vi "Append Ring StringsAndValues.vi"(8 "error in (no error)":errorcluster, 9 "Value":i32, 10 "String":string, 11 "Ring in":refnum<vi>) -> (0 "error out":errorcluster, 2 "StringsAndValues[]":T1, 3 "Ring out":refnum<vi>)   [LabVIEW 2019, in "Control Experiment.lvclass"]
uses:
  Control Experiment.lvclass
  <vilib>/Utility/miscctls.llb/LVStringsAndValuesArrayTypeDef.ctl
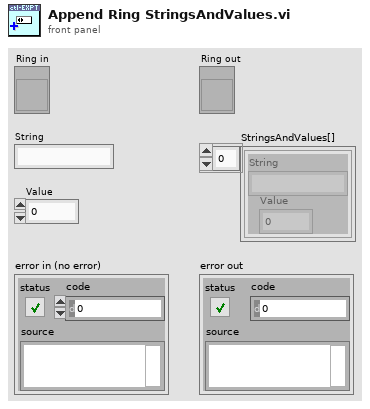
[diagram p1: front panel]
types:
  T1 = typedef "LVStringsAndValuesArrayTypeDef.ctl" = cluster{"String":string, "Value":ext}[]
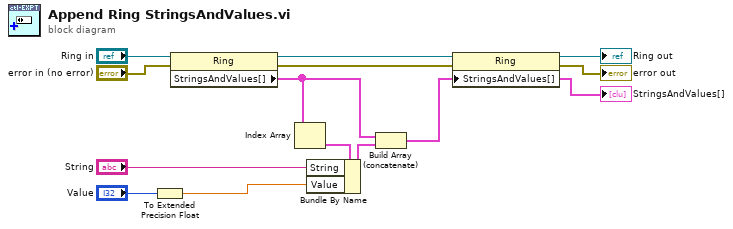
[diagram p0: block diagram]
diagram:
  n1 = To Extended Precision Float(1:"Value") -> (0:w4:ext)
  n2 = property class="Ring"(reference="Ring in", error in="error in (no error)") -> (reference out=w6:refnum<vi>, error out=w7:errorcluster, "StringsAndValues[]"=w2:T1)
  n3 = Index Array(array=w2) -> (element=w8:cluster{"String":string, "Value":ext})  [unwired: 1 in]
  n4 = Bundle By Name(cluster=w8, "String"="String", "Value"=w4) -> (w3:cluster{"String":string, "Value":ext})
  n5 = Build Array (concatenate)(w2, w3) -> (w1:T1)
  "StringsAndValues[]" <- w1
  n6 = property class="Ring"(reference=w6, error in=w7, "StringsAndValues[]"=w1) -> (reference out=→"Ring out":refnum<vi>, error out=→"error out":errorcluster)
